vi "cluster_test.vi"() -> ()   [LabVIEW 2010]
panel:
  out "Cluster":cluster{"some crap":dbl, "the num 2":dbl}
  in  "some crap":dbl
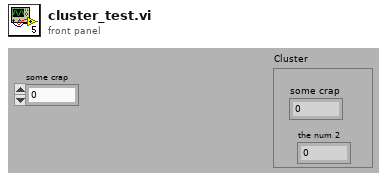
[diagram p1: front panel]
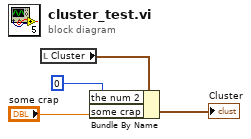
[diagram p0: block diagram]
diagram:
  n1 = local read "Cluster"() -> (w1:cluster{"some crap":dbl, "the num 2":dbl})
  n2 = Bundle By Name(cluster=w1, "the num 2"=0, "some crap"="some crap") -> (→"Cluster":cluster{"some crap":dbl, "the num 2":dbl})
